vi "2015Swerve_SteeringAdjustment_v2.vi"(8 "Encoder Ticks Per Rev":dbl=1988.0, 9 "Wheel Power":dbl, 10 "Encoder Setpoint":dbl, 11 "Encoder Position":dbl) -> (1 "Wheel Power Out":dbl, 2 "Encoder Setpoint Out":dbl)   [LabVIEW 2014]
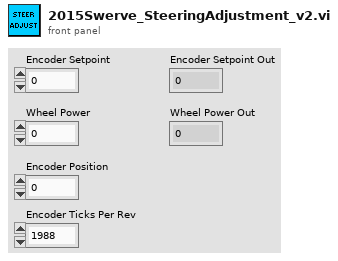
[diagram p1: front panel]
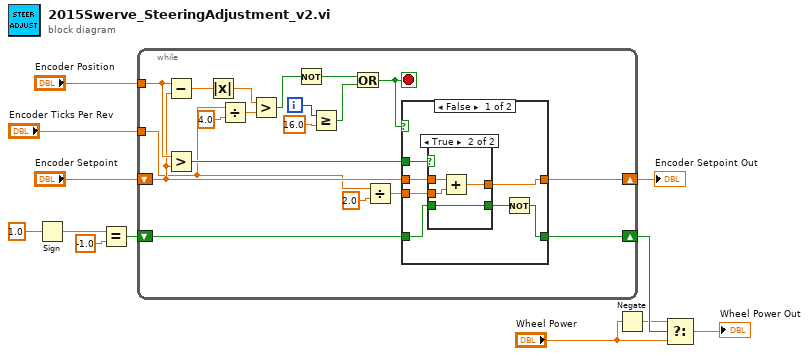
[diagram p0: block diagram]
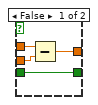
[diagram p2: hidden frame]
diagram:
  n1 = Sign(1:1.0 ("number")) -> (0:w5:dbl)
  n2 = Equal?(x=w5, y=-1.0) -> (x = y?=w3:bool)
  n3 = while {
    tunnel: "Encoder Position" -> [w22]
    shift-right: [w28] -> w12
    shift-left: "Encoder Setpoint" -> [w21]
    shift-right: [w19] -> w11
    shift-left: w3 -> [w18]
    tunnel: "Encoder Ticks Per Rev" -> [w14]
    i -> [w29]
    stop <- w20 stop-if-true
    n4 = Subtract(x=w22, y=w21) -> (x-y=w27:dbl)
    n5 = Greater?(x=w22, y=w21) -> (0:w23:bool)
    n6 = Absolute Value(x=w27) -> (abs(x)=w26:dbl)
    n7 = Divide(x=w14, y=4.0) -> (x/y=w16:dbl)
    n8 = Greater?(x=w26, y=w16) -> (0:w25:bool)
    n9 = Not(x=w25) -> (.not. x?=w24:bool)
    n10 = Greater Or Equal?(x=w29, y=16.0) -> (x >= y?=w31:bool)
    n11 = Or(x=w24, y=w31) -> (x .or. y?=w20:bool)
    n12 = Divide(x=w14, y=2.0) -> (x/y=w13:dbl)
    n13 = case shown="False" w20 {
      tunnel: [w38 w48] -> w28
      tunnel: w23 -> [w37 _]
      tunnel: w21 -> [w36 w48]
      tunnel: [w33 w47] -> w19
      tunnel: w18 -> [w34 w47]
      tunnel: w13 -> [w32 _]
      frame False {
        n14 = case shown="True" w37 {
          tunnel: w36 -> [w42 w46]
          tunnel: [w41 w45] -> w38
          tunnel: [w40 w44] -> w35
          tunnel: w34 -> [w40 w44]
          tunnel: w32 -> [w39 w43]
          frame False {
            n15 = Subtract(x=w42, y=w39) -> (x-y=w41:dbl)
          }
          frame True {
            n16 = Add(x=w46, y=w43) -> (x+y=w45:dbl)
          }
        }
        n17 = Not(x=w35) -> (.not. x?=w33:bool)
      }
      frame True {
      }
    }
  }
  "Encoder Setpoint Out" <- w12
  n18 = Negate(x="Wheel Power") -> (-x=w10:dbl)
  n19 = Select(t=w10, s=w11, f="Wheel Power") -> (s? t:f=→"Wheel Power Out":dbl)
